vi "Snap 90__Foreward.vi"(9 "YawWrap":dbl) -> (1 "Snap Goal":dbl=-90.0, 2 "Backwards?":bool)   [LabVIEW 2018]
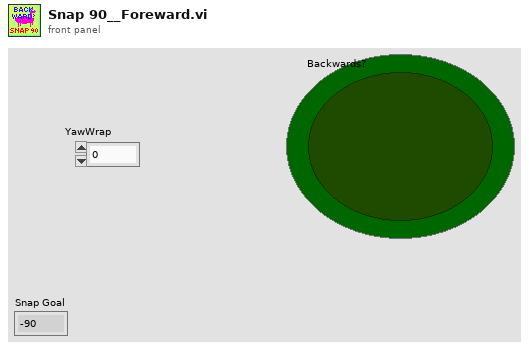
[diagram p1: front panel]
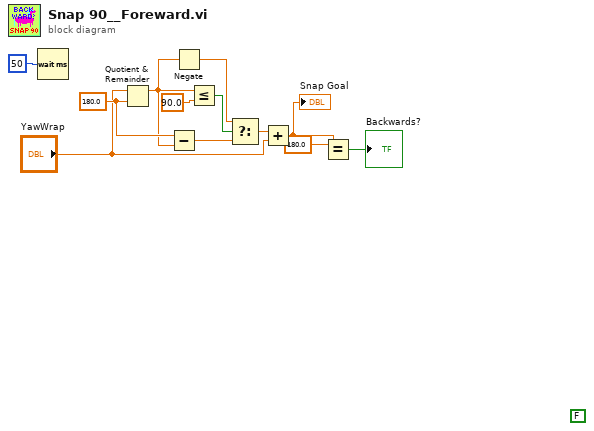
[diagram p0: block diagram]
diagram:
  (unwired) FALSE
  w10 = 180.0 ("y")
  n1 = Wait (ms)(milliseconds to wait=u32 50) -> ()  [unwired: 1 out]
  n2 = Quotient & Remainder(x="YawWrap", y=w10) -> (x-y*floor(x/y)=w9:dbl)  [unwired: 1 out]
  n3 = Subtract(x=w10, y=w9) -> (x-y=w8:dbl)
  n4 = Negate(x=w9) -> (-x=w12:dbl)
  n5 = Less Or Equal?(x=w9, y=90.0) -> (x <= y?=w6:bool)
  n6 = Select(t=w12, s=w6, f=w8) -> (s? t:f=w11:dbl)
  n7 = Add(x=w11, y="YawWrap") -> (x+y=w3:dbl)
  "Snap Goal" <- w3
  n8 = Equal?(x=180.0, y=w3) -> (x = y?=→"Backwards?":bool)
